vi "Credito Reset MXN.vi"(8 "error in (no error)":errorcluster, 11 "MXN actor in":refnum<class "MXN actor.lvclass">) -> (0 "error out":errorcluster, 3 "MXN actor out":refnum<class "MXN actor.lvclass">)   [LabVIEW 2020, in "MXN actor.lvlib" / "MXN actor.lvclass"]
uses:
  MXN actor.lvclass
  MXN actor.lvclass/MXN actor.ctl
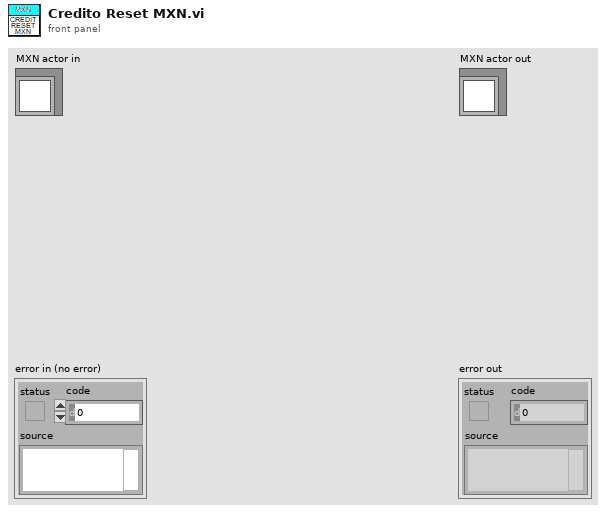
[diagram p1: front panel]
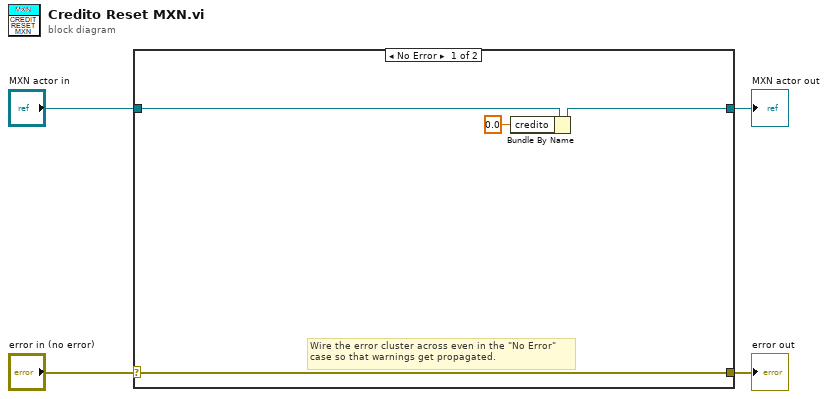
[diagram p0: block diagram]
diagram:
  n1 = case shown="No Error" "error in (no error)" {
    selector: "error in (no error)" -> [w7 w10]
    tunnel: [w7 w10] -> w3
    tunnel: [w6 w9] -> w1
    tunnel: "MXN actor in" -> [w8 w9]
    frame No Error {
      # "Wire the error cluster across even in the \"No Error\"\ncase so that warnings get propagated."
      n2 = Bundle By Name(cluster=w8, "credito"=0.0) -> (w6:refnum<class "MXN actor.lvclass">)
    }
    frame Error {
    }
  }
  "error out" <- w3
  "MXN actor out" <- w1
